vi "catch_block_in_body.vi"(8 "error in 2":errorcluster, 11 "KNR in 3":T1) -> (0 "error out 4":errorcluster, 3 "KNR out 4":T1)   [LabVIEW 2013]
uses:
  <userlib>/KNR OS 3.0 LabVIEW Toolkit/Type Definition/KNR3 Reference.ctl
  <userlib>/_FPGA Interface Advanced Tools/FPGA Interface Base/FPGA Interface Base.lvclass
  <userlib>/KNR OS 3.0 LabVIEW Toolkit/Type Definition/Resource.ctl
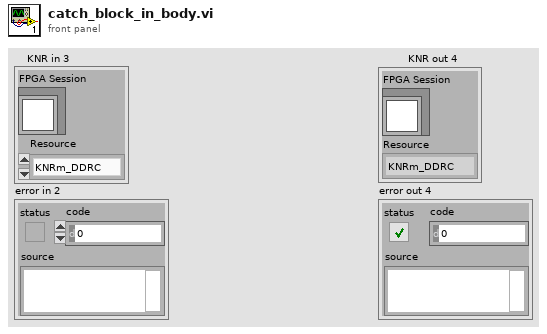
[diagram p1: front panel]
types:
  T1 = typedef "KNR3 Reference.ctl" = cluster{"FPGA Session":refnum<class "FPGA Interface Base.lvclass">, "Resource":T2}
  T2 = typedef "Resource.ctl" = enum16{"KNRm_DDRC", "KNRm_DDDD", "KNRm_DDDR", "KNRm_DDDC", "KNR"}
  T3 = cluster{"Mode":enum16{"FRWD", "TURFIX", "TURNOF"}, "Dir":enum16{"Left", "Right"}, "Pcmd":dbl, "Vcmd":dbl}
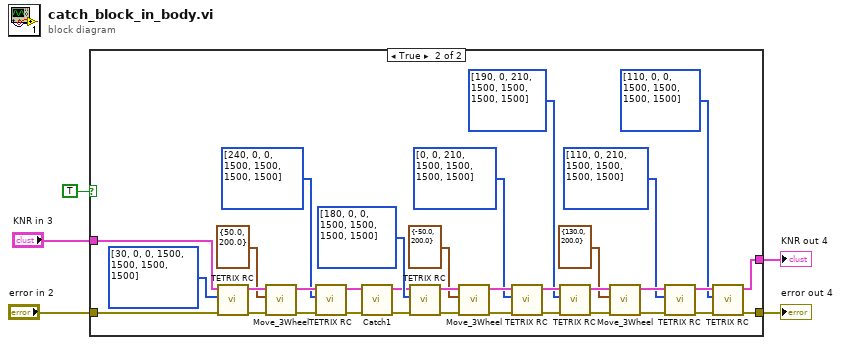
[diagram p0: block diagram]
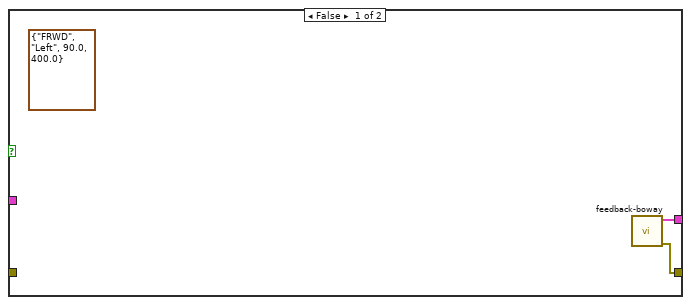
[diagram p2: hidden frame]
diagram:
  n1 = case shown="True" TRUE {
    tunnel: [w7 w10] -> w1
    tunnel: [w6 w11] -> w2
    tunnel: "KNR in 3" -> [_ w9]
    tunnel: "error in 2" -> [_ w8]
    frame False {
      (unwired) T3 {"Mode"=enum."FRWD", "Dir"=enum."Left", "Pcmd"=90.0, "Vcmd"=400.0} ("Move")
      n2 = call "feedback-boway.vi"() -> ("error out"=w7:errorcluster, "KNR out"=w6:T1)  [unwired: 9 in, 1 out]
    }
    frame True {
      n3 = call "TETRIX RC.vi"("error in 2"=w8, "RC"=u16[] [30, 0, 0, 1500, 1500, 1500, 1500], "KNR in 3"=w9) -> ("error out 4"=w39:errorcluster, "KNR out 4"=w40:T1)  [unwired: 7 in]
      n4 = call "Move_3Wheel.vi"("error in (no error)"=w39, "Cluster"=cluster{"UDmm)":dbl, "Vcmd":dbl} {"UDmm)"=50.0, "Vcmd"=200.0}, "KNR in"=w40) -> ("error out"=w36:errorcluster, "KNR out"=w37:T1)  [unwired: 7 in]
      n5 = call "TETRIX RC.vi"("error in 2"=w36, "RC"=u16[] [240, 0, 0, 1500, 1500, 1500, 1500], "KNR in 3"=w37) -> ("error out 4"=w20:errorcluster, "KNR out 4"=w21:T1)  [unwired: 7 in]
      n6 = call "Catch1.vi"("Error"=w20, "KNR in"=w21) -> ("error out 4"=w18:errorcluster, "KNR out"=w19:T1)  [unwired: 6 in, 2 out]
      n7 = call "TETRIX RC.vi"("error in 2"=w18, "RC"=u16[] [180, 0, 0, 1500, 1500, 1500, 1500], "KNR in 3"=w19) -> ("error out 4"=w32:errorcluster, "KNR out 4"=w33:T1)  [unwired: 7 in]
      n8 = call "Move_3Wheel.vi"("error in (no error)"=w32, "Cluster"=cluster{"UDmm)":dbl, "Vcmd":dbl} {"UDmm)"=-50.0, "Vcmd"=200.0}, "KNR in"=w33) -> ("error out"=w29:errorcluster, "KNR out"=w30:T1)  [unwired: 7 in]
      n9 = call "TETRIX RC.vi"("error in 2"=w29, "RC"=u16[] [0, 0, 210, 1500, 1500, 1500, 1500], "KNR in 3"=w30) -> ("error out 4"=w26:errorcluster, "KNR out 4"=w27:T1)  [unwired: 7 in]
      n10 = call "TETRIX RC.vi"("error in 2"=w26, "RC"=u16[] [190, 0, 210, 1500, 1500, 1500, 1500], "KNR in 3"=w27) -> ("error out 4"=w24:errorcluster, "KNR out 4"=w23:T1)  [unwired: 7 in]
      n11 = call "Move_3Wheel.vi"("error in (no error)"=w24, "Cluster"=cluster{"UDmm)":dbl, "Vcmd":dbl} {"UDmm)"=130.0, "Vcmd"=200.0}, "KNR in"=w23) -> ("error out"=w16:errorcluster, "KNR out"=w17:T1)  [unwired: 7 in]
      n12 = call "TETRIX RC.vi"("error in 2"=w16, "RC"=u16[] [110, 0, 210, 1500, 1500, 1500, 1500], "KNR in 3"=w17) -> ("error out 4"=w14:errorcluster, "KNR out 4"=w13:T1)  [unwired: 7 in]
      n13 = call "TETRIX RC.vi"("error in 2"=w14, "RC"=u16[] [110, 0, 0, 1500, 1500, 1500, 1500], "KNR in 3"=w13) -> ("error out 4"=w10:errorcluster, "KNR out 4"=w11:T1)  [unwired: 7 in]
    }
  }
  "KNR out 4" <- w2
  "error out 4" <- w1
